vi "Read Database.vi"(8 "error in":errorcluster, 11 "Path":path=path "C:/dev/niveristand-communications-bus-template/Source/Databases/DB_2F_Test.json") -> (0 "error out":errorcluster, 2 "Database":T1)   [LabVIEW 2020, in "Communication Bus Template System Explorer.lvlib"]
doc: "This VI reads a simple json database file that includes a Baud Rate and Frames where each frame includes a Name and ID."
uses:
  Communication Bus Template System Explorer.lvlib
  Types/Database.ctl
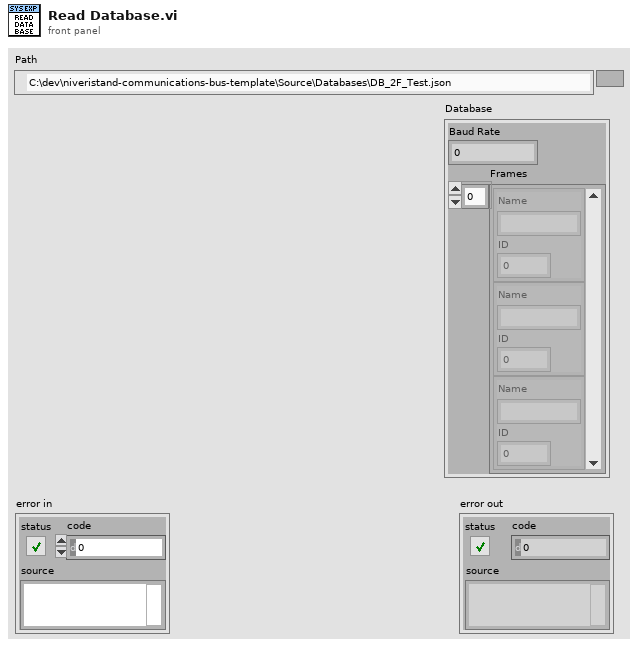
[diagram p1: front panel]
types:
  T1 = typedef "Communication Bus Template System Explorer.lvlib/Database.ctl" = cluster{"Baud Rate":u64, "Frames":cluster{"Name":string, "ID":i32}[]}
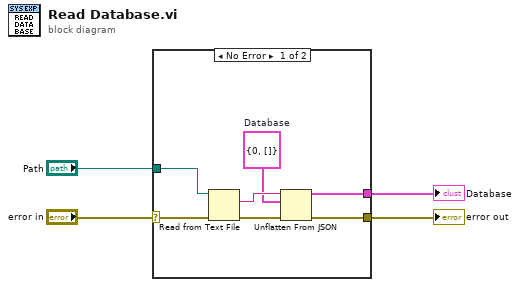
[diagram p0: block diagram]
diagram:
  n1 = case shown="No Error" "error in" {
    selector: "error in" -> [w10 w12]
    tunnel: "Path" -> [w11 _]
    tunnel: [w6 w12] -> w2
    tunnel: [w5 _] -> w1
    frame No Error {
      w7 = T1 {"Baud Rate"=0, "Frames"=[]}  # Database
      n2 = Read from Text File(file (use dialog)=w11, error in=w10) -> (text=w8:string, error out=w9:errorcluster)  [unwired: 2 in, 2 out]
      n3 = Unflatten From JSON(JSON string=w8, type and defaults=w7, error in (no error)=w9) -> (value=w5:T1, error out=w6:errorcluster)  [unwired: 4 in]
    }
    frame Error {
    }
  }
  "Database" <- w1
  "error out" <- w2
